vi "CRYUpdate Steps Input Control.vi"   [LabVIEW 2013]
uses:
  CRYStepSetup/CRYStepSetup Global.vi
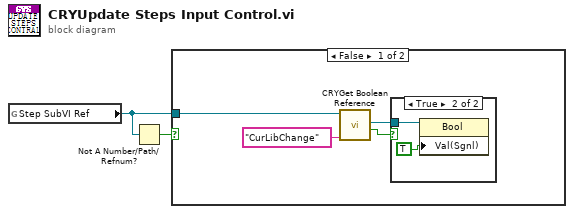
[diagram p0: block diagram]
diagram:
  n1 = global read "CRYStepSetup Global.vi" "Step SubVI Ref"() -> (w2:refnum<vi>)
  n2 = Not A Number/Path/Refnum?(number/path/refnum=w2) -> (NaN/Path/Refnum?=w1:bool)
  n3 = case shown="False" w1 {
    tunnel: w2 -> [w6 _]
    frame False {
      n4 = call "CRYGet Boolean Reference.vi"("Label Name"="CurLibChange" ("Label.Text"), "VI Refnum"=w6) -> ("Exist?"=w3:bool, "Boolean Ref"=w5:refnum<vi>)  [unwired: 8 out]
      n5 = case shown="True" w3 {
        tunnel: w5 -> [_ w8]
        frame False {
        }
        frame True {
          n6 = property class="Bool"(reference=w8, "Val(Sgnl)"=TRUE ("NewVal")) -> ()  [unwired: 1 in, 2 out]
        }
      }
    }
    frame True {
    }
  }
